vi "BK Precision 9200 Series Create and Save List Program.vi"() -> ()   [LabVIEW 2021]
doc: "This example demonstrates how to create a simple list program by storing values of steps from arrays."
uses:
  <instrlib>/BK Precision 9200 Series/BK Precision 9200 Series.lvlib
panel:
  in  "Step Time":dbl[](array[numeric])=[1.0, 1.0, 1.0, 1.0, 1.0, 1.0, 1.0, 1.0, 1.0, 1.0] min=0.001 max=65.535 step=0.001 format="%.3f"
  in  "Step Current":dbl[](array[numeric])=[1.0, 1.0, 1.0, 1.0, 1.0, 1.0, 1.0, 1.0, 1.0, 1.0] min=0.0 max=25.0 step=1.0 format="%.4f"
  in  "Step Voltage":dbl[](array[numeric])=[1.0, 1.0, 1.0001, 1.0001, 1.0, 1.0, 1.0, 1.0, 1.0, 1.0001] min=0.0 max=150.0 step=1.0 format="%.3f"
  in  "VISA resource name":refnum<visa-resource-name>
  # "(c) 2014 B&K Precision Corporation.  ALL RIGHTS RESERVED."
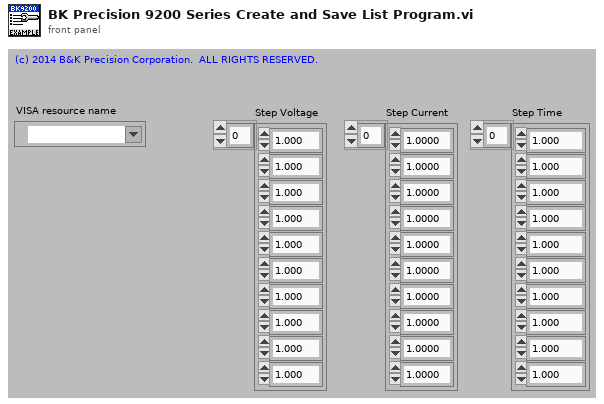
[diagram p1: front panel]
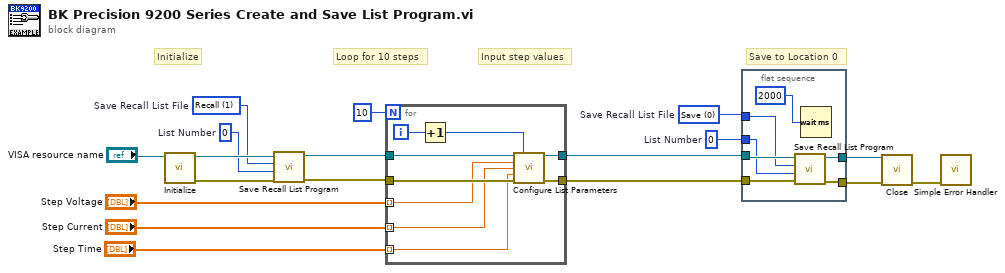
[diagram p0: block diagram]
diagram:
  w1 = u16 0 items=["Save", "Recall"]  # Save Recall List File
  w2 = 0  # List Number
  w3 = u16 1 items=["Save", "Recall"]  # Save Recall List File
  w4 = 0  # List Number
  # "Save to Location 0"
  # "Loop for 10 steps"
  # "Input step values"
  # "Initialize"
  n1 = call <instrlib>:"Initialize.vi"("VISA resource name"="VISA resource name") -> ("error out"=w7:errorcluster, "VISA resource name out"=w8:refnum<visa-resource-name>)  [unwired: 9 in]
  n2 = call <instrlib>:"Save Recall List Program.vi"("error in (no error)"=w7, "List Number (0)"=w2, "Save Recall List File (0:Save)"=w3, "VISA resource name"=w8) -> ("error out"=w6:errorcluster, "VISA resource name out"=w5:refnum<visa-resource-name>)  [unwired: 6 in]
  n3 = for {
    N: 10 -> [_]
    tunnel: "Step Voltage" -> [w23] mode=indexing
    tunnel: "Step Current" -> [w22] mode=indexing
    tunnel: "Step Time" -> [w21] mode=indexing
    tunnel: w5 -> [w25]
    tunnel: [w26] -> w12
    tunnel: w6 -> [w27]
    tunnel: [w24] -> w9
    i -> [w20]
    n4 = Increment(x=w20) -> (x+1=w19:i32)
    n5 = call <instrlib>:"Configure List Parameters.vi"("VISA resource name"=w25, "Step Number (1)"=w19, "Step Voltage (1.000)"=w23, "Step Current (1.0000)"=w22, "Step Time (1)"=w21, "error in (no error)"=w27) -> ("VISA resource name out"=w26:refnum<visa-resource-name>, "error out"=w24:errorcluster)  [unwired: 8 in]
  }
  n6 = flat-sequence {
    tunnel: w12 -> [w32]
    tunnel: w9 -> [w33]
    tunnel: [w31] -> w11
    tunnel: [w30] -> w10
    tunnel: w1 -> [w29]
    tunnel: w4 -> [w28]
    frame #0 {
      n7 = call <instrlib>:"Save Recall List Program.vi"("error in (no error)"=w33, "List Number (0)"=w28, "Save Recall List File (0:Save)"=w29, "VISA resource name"=w32) -> ("error out"=w30:errorcluster, "VISA resource name out"=w31:refnum<visa-resource-name>)  [unwired: 6 in]
      n8 = Wait (ms)(milliseconds to wait=2000) -> ()  [unwired: 1 out]
    }
  }
  n9 = call <instrlib>:"Close.vi"("error in (no error)"=w10, "VISA resource name"=w11) -> ("error out"=w17:errorcluster)  [unwired: 9 in]
  n10 = call <vilib>:"Simple Error Handler.vi"("error in (no error)"=w17) -> ()  [unwired: 4 in, 5 out]
